vi "get daemons.vi"(8 "error in":errorcluster, 11 "module in":refnum<class "TBM module execution interface.lvclass">) -> (0 "error out":errorcluster, 2 "daemons":refnum<vi>[](array[refnum]), 3 "module out":refnum<class "TBM module execution interface.lvclass">)   [LabVIEW 2013, in "TBM module execution interface.lvclass"]
uses:
  TBM module execution interface.lvclass
  <vilib>/NI/Tag Bus/data stream/publisher/publisher.lvclass
  <vilib>/NI/Tag Bus/data stream/subscriber/subscriber.lvclass
  stream daemon template.vi
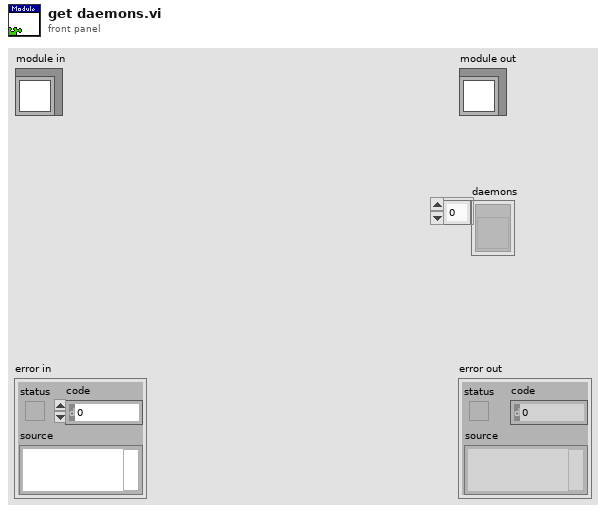
[diagram p1: front panel]
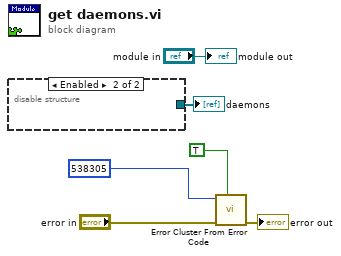
[diagram p0: block diagram]
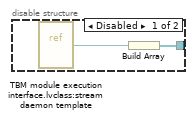
[diagram p2: hidden frame]
diagram:
  n1 = disable-structure shown="Enabled" {
    disable-tunnel: [w7 _] -> w1
    frame Disabled {
      n2 = vi-ref "TBM module execution interface.lvclass:stream daemon template.vi"() -> (w8:refnum<vi>)
      n3 = Build Array(w8) -> (w7:refnum<vi>[])
    }
    frame Enabled {
    }
  }
  "daemons" <- w1
  n4 = call <vilib>:"Error Cluster From Error Code.vi"("show call chain? (False)"=TRUE, "error in (no error)"="error in", "error code (0)"=538305) -> ("error out"=→"error out":errorcluster)  [unwired: 6 in]
  "module out" <- "module in"
